vi "Commands array generator.vi"(4 "Axis 1":string, 6 "Axis in":string, 8 "Axes speed \n(µm/s)":i32, 9 "Y Step size in µm":i32, 10 "T/F product array":bool[][](array[boolean]), 11 "Space defined array":dbl[][](array[numeric])) -> (2 "Command Array":string[][](array[string]), 3 "Time Array":dbl[][](array[numeric]))   [LabVIEW 2016]
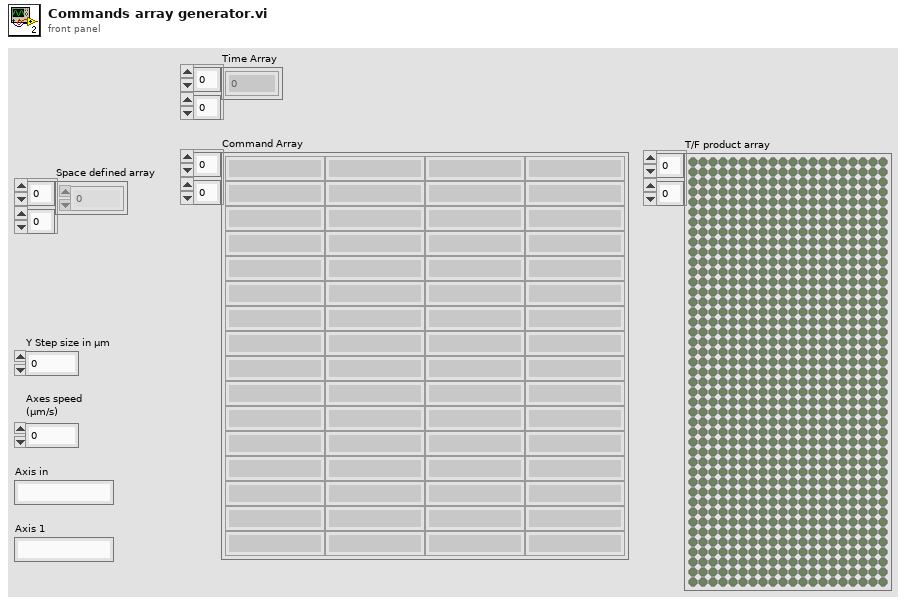
[diagram p1: front panel]
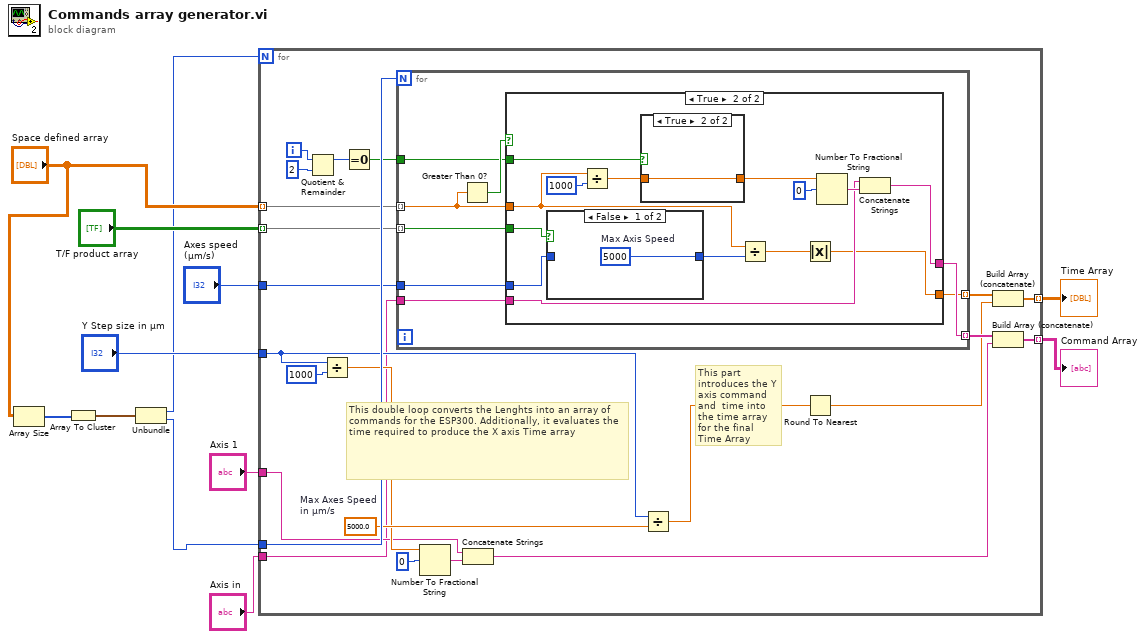
[diagram p0: block diagram]
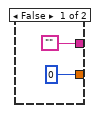
[diagram p2: hidden frame]
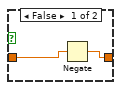
[diagram p4: hidden frame]
diagram:
  n1 = Array Size(array="Space defined array") -> (size(s)=w4:i32[])
  n2 = Array To Cluster(array=w4) -> (cluster=w5:cluster{"[0]":i32, "[1]":i32})
  n3 = Unbundle(w5) -> ("[0]"=w2:i32, "[1]"=w1:i32)
  n4 = for {
    N: w2 -> [_]
    tunnel: w1 -> [w35]
    tunnel: "Space defined array" -> [w34] mode=indexing
    tunnel: [w31] -> w7 mode=indexing
    tunnel: "T/F product array" -> [w24] mode=indexing
    tunnel: [w21] -> w8 mode=indexing
    tunnel: "Y Step size in µm" -> [w16]
    tunnel: "Axis 1" -> [w15]
    tunnel: "Axis in" -> [w14]
    tunnel: "Axes speed \n(µm/s)" -> [w13]
    i -> [w26]
    w20 = 5000.0  # Max Axes Speed in µm/s
    # "This part introduces the Y axis command and  time into the time array for the final Time Array"
    # "This double loop converts the Lenghts into an array of commands for the ESP300. Additionally, it evaluates the time required to produce the X axis Time array"
    n5 = Quotient & Remainder(x=w26, y=2) -> (x-y*floor(x/y)=w28:i32)  [unwired: 1 out]
    n6 = Divide(x=w16, y=1000) -> (x/y=w19:dbl)
    n7 = Equal To 0?(x=w28) -> (x = 0?=w25:bool)
    n8 = for {
      N: w35 -> [_]
      tunnel: w34 -> [w43] mode=indexing
      tunnel: [w41] -> w30 mode=indexing
      tunnel: w25 -> [w40]
      tunnel: [w39] -> w22 mode=indexing
      tunnel: w24 -> [w38] mode=indexing
      tunnel: w14 -> [w37]
      tunnel: w13 -> [w36]
      n9 = Greater Than 0?(x=w43) -> (x > 0?=w42:bool)
      n10 = case shown="True" w42 {
        tunnel: w43 -> [_ w53]
        tunnel: ["" w58] -> w41
        tunnel: w40 -> [_ w56]
        tunnel: [0 w46] -> w39
        tunnel: w38 -> [_ w51]
        tunnel: w37 -> [_ w48]
        tunnel: w36 -> [_ w47]
        frame False {
        }
        frame True {
          n11 = case shown="False" w51 {
            tunnel: [w60 w61] -> w52
            tunnel: w47 -> [_ w61]
            frame False {
              w60 = 5000  # Max Axis Speed
            }
            frame True {
            }
          }
          n12 = Divide(x=w53, y=1000) -> (x/y=w54:dbl)
          n13 = case shown="True" w56 {
            tunnel: w54 -> [w63 w64]
            tunnel: [w62 w64] -> w55
            frame False {
              n14 = Negate(x=w63) -> (-x=w62:dbl)
            }
            frame True {
            }
          }
          n15 = Divide(x=w53, y=w52) -> (x/y=w49:dbl)
          n16 = Absolute Value(x=w49) -> (abs(x)=w46:dbl)
          n17 = Number To Fractional String(number=w55, width (-)=i16 0) -> (F-format string=w50:string)  [unwired: 2 in]
          n18 = Concatenate Strings(w48, w50) -> (w58:string)
        }
      }
    }
    n19 = Number To Fractional String(number=w19, width (-)=i16 0) -> (F-format string=w23:string)  [unwired: 2 in]
    n20 = Concatenate Strings(w15, w23) -> (w32:string)
    n21 = Divide(x=w16, y=w20) -> (x/y=w18:dbl)
    n22 = Round To Nearest(number=w18) -> (nearest integer value=w17:dbl)
    n23 = Build Array (concatenate)(w22, w17) -> (w21:dbl[])
    n24 = Build Array (concatenate)(w30, w32) -> (w31:string[])
  }
  "Time Array" <- w8
  "Command Array" <- w7
